vi "max_min_hold (SubVI).vi"(11 "theta":dbl) -> (2 "theta_min":dbl, 3 "theta_max":dbl)   [LabVIEW 2013]
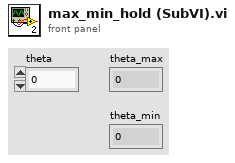
[diagram p1: front panel]
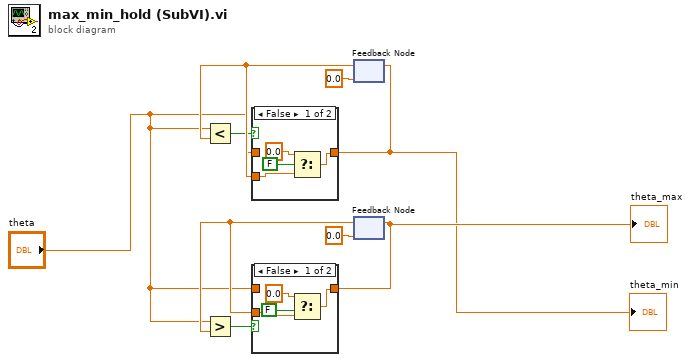
[diagram p0: block diagram]
diagram:
  n1 = feedback #1 ("Feedback Node 2")(0.0 ("Value 2")) -> (w7:dbl)
  n2 = Less?(x="theta", y=w7) -> (x < y?=w6:bool)
  n3 = case "Case Structure 2" shown="False" w6 {
    tunnel: "theta" -> [_ w14]
    tunnel: [w13 w14] -> w1
    tunnel: w7 -> [w11 _]
    frame False {
      n4 = Select ("Select 2")(t=0.0 ("t 2"), s=FALSE, f=w11) -> (s? t:f=w13:dbl)
    }
    frame True {
    }
  }
  "theta_min" <- w1
  n5 = feedback-in #1 ("3")(w1) -> ()
  n6 = feedback #2(0.0 ("Value")) -> (w8:dbl)
  n7 = Greater?(x="theta", y=w8) -> (0:w9:bool)
  n8 = case shown="False" w9 {
    tunnel: "theta" -> [_ w19]
    tunnel: [w18 w19] -> w2
    tunnel: w8 -> [w16 _]
    frame False {
      n9 = Select(t=0.0, s=FALSE, f=w16) -> (s? t:f=w18:dbl)
    }
    frame True {
    }
  }
  "theta_max" <- w2
  n10 = feedback-in #2 ("2")(w2) -> ()
